vi "test_OpenClose (lowLevel).vi"() -> ()   [LabVIEW 2020]
uses:
  <instrlib>/AIM GmbH/_AIM 664/AIM664LV.lvlib
  <instrlib>/AIM GmbH/_AIM 664/bsp/Fdx Create Session (Tx-UDP Port-Oriented).vi
panel:
  out "instances count 4":i32
  in  "finalize":bool=TRUE
  out "instances count 3":i32
  out "instances count 2":i32
  out "instances count":i32
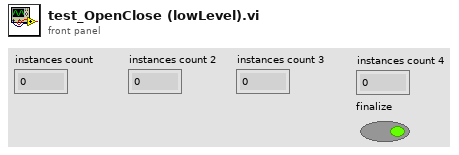
[diagram p1: front panel]
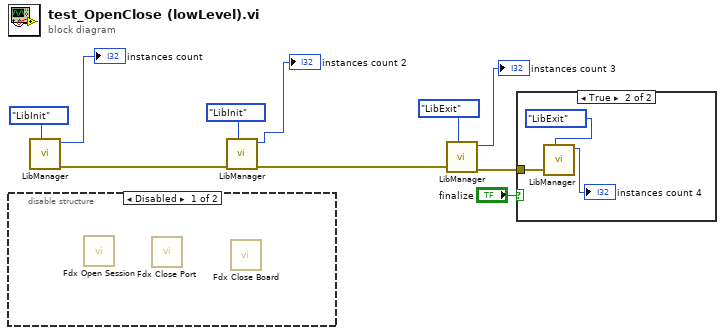
[diagram p0: block diagram]
diagram:
  n1 = disable-structure shown="Disabled" {
    frame Disabled {
      n2 = call-poly <instrlib>:"Fdx Open Session.vi"() -> ()  [unwired: 7 in, 5 out]
      n3 = call <instrlib>:"Fdx Close Port.vi"() -> ()  [unwired: 10 in, 2 out]
      n4 = call <instrlib>:"Fdx Close Board.vi"() -> ()  [unwired: 11 in, 1 out]
    }
    frame Enabled {
    }
  }
  n5 = call <instrlib>:"LibManager.vi"("action"=enum16{"LibInit", "LibExit"}."LibInit") -> ("error out"=w10:errorcluster, "instances count"=→"instances count":i32)  [unwired: 8 in, 1 out]
  n6 = call <instrlib>:"LibManager.vi"("action"=enum16{"LibInit", "LibExit"}."LibInit", "error in (no error)"=w10) -> ("error out"=w4:errorcluster, "instances count"=→"instances count 2":i32)  [unwired: 7 in, 1 out]
  n7 = call <instrlib>:"LibManager.vi"("action"=enum16{"LibInit", "LibExit"}."LibExit", "error in (no error)"=w4) -> ("error out"=w2:errorcluster, "instances count"=→"instances count 3":i32)  [unwired: 7 in, 1 out]
  n8 = case shown="True" "finalize" {
    tunnel: w2 -> [_ w13]
    frame False {
    }
    frame True {
      n9 = call <instrlib>:"LibManager.vi"("action"=enum16{"LibInit", "LibExit"}."LibExit", "error in (no error)"=w13) -> ("instances count"=→"instances count 4":i32)  [unwired: 7 in, 2 out]
    }
  }
